vi "Pick Point.vi"(7 "Actual Transform In":T1, 8 "error in (no error)":errorcluster, 9 "Coords":cluster{"Horizontal":i32, "Vertical":i32}, 10 "Vertex Array":cluster{"X":sgl, "Y":sgl, "Z":sgl}[](array[cluster]), 11 "3D Picture Control In":refnum<vi>) -> (0 "error out":errorcluster, 1 "Hit Any Point?":bool, 2 "Snap Cursor Position":cluster{"X":sgl, "Y":sgl, "Z":sgl}, 3 "3D Picture Control Out":refnum<vi>, 5 "Actual Transform Out":T1)   [LabVIEW 2020, in "3D Plot.lvclass"]
uses:
  3D Plot.lvclass
  Actual Transform.ctl
  Range Clusters.ctl
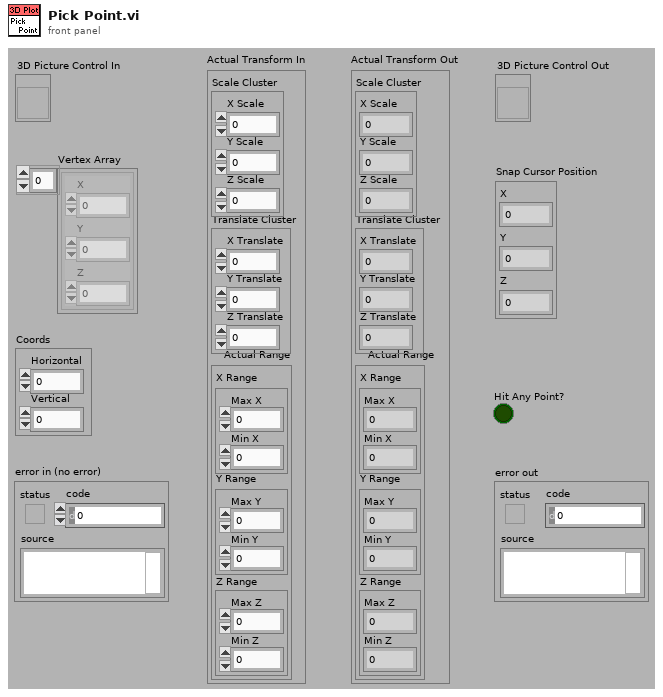
[diagram p1: front panel]
types:
  T1 = typedef "3D Plot.lvclass/Actual Transform.ctl" = cluster{"Scale Cluster":cluster{"X Scale":sgl, "Y Scale":sgl, "Z Scale":sgl}, "Translate Cluster":cluster{"X Translate":sgl, "Y Translate":sgl, "Z Translate":sgl}, "Actual Range":T2}
  T2 = typedef "3D Plot.lvclass/Range Clusters.ctl" = cluster{"X Range":cluster{"Max X":sgl, "Min X":sgl}, "Y Range":cluster{"Max Y":sgl, "Min Y":sgl}, "Z Range":cluster{"Max Z":sgl, "Min Z":sgl}}
  T3 = cluster{"Real Matrix Element":sgl, "Real Matrix Element":sgl, "Real Matrix Element":sgl}[]
  T4 = cluster{"Real Matrix Element":sgl, "Real Matrix Element":sgl, "Real Matrix Element":sgl}
  T5 = typedef "LVPoint32TypeDef.ctl" = cluster{"Horizontal":i32, "Vertical":i32}
  T6 = typedef "LVBoundsTypeDef.ctl" = cluster{"Width":u32, "Height":u32}
  T7 = cluster{"Product[0]":sgl, "Product[1]":sgl, "Product[2]":sgl}
  T8 = cluster{"X Translate":sgl, "Y Translate":sgl, "Z Translate":sgl}
  T9 = cluster{"X Scale":sgl, "Y Scale":sgl, "Z Scale":sgl}
  T10 = cluster{cluster{"Product[0]":sgl, "Product[1]":sgl, "Product[2]":sgl}, cluster{"Product[0]":sgl, "Product[1]":sgl, "Product[2]":sgl}}
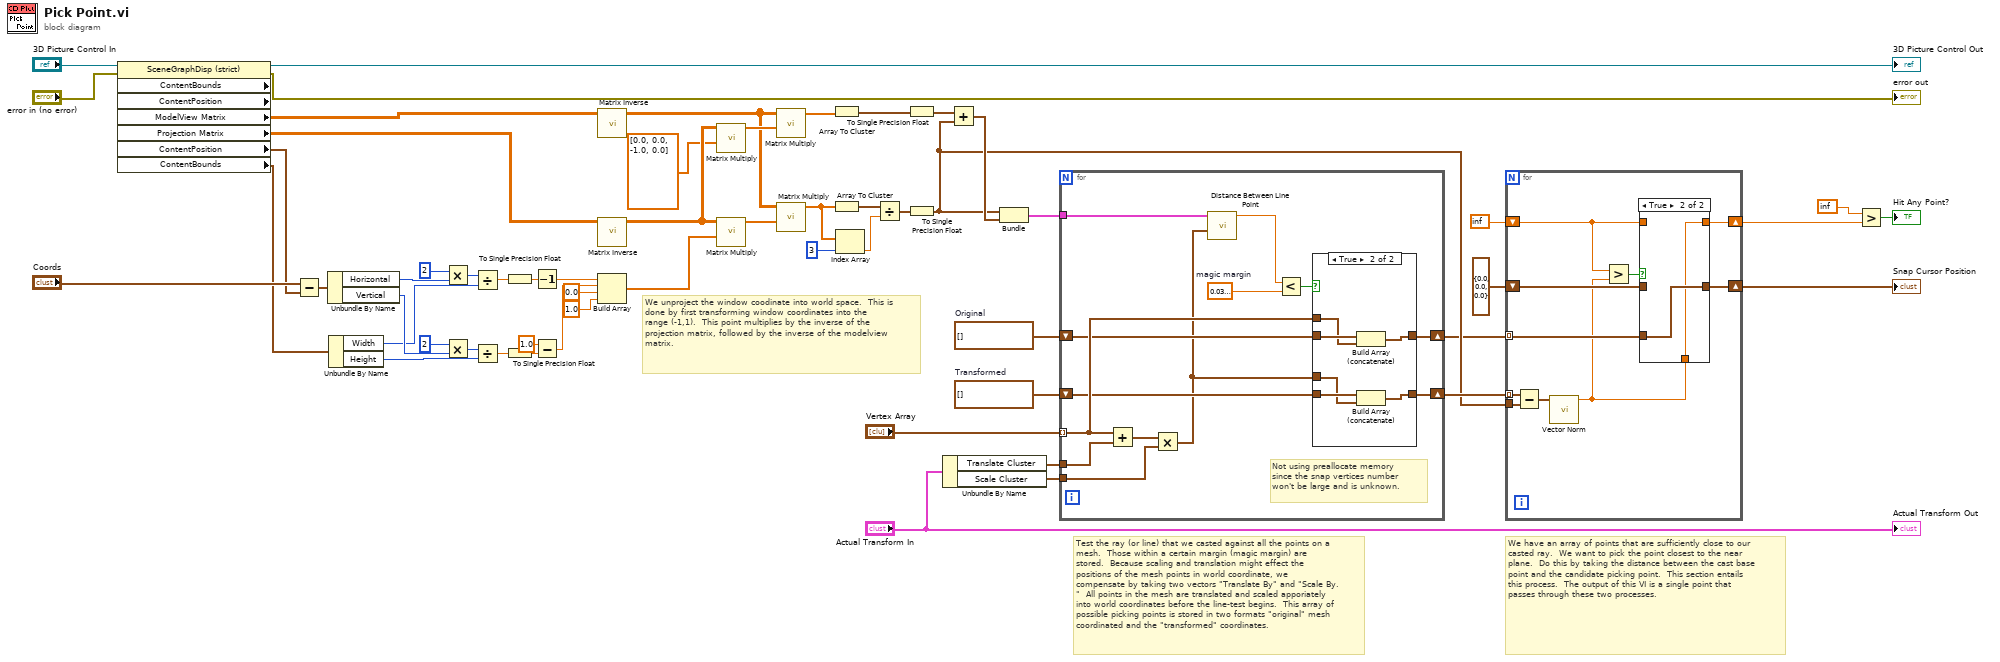
[diagram p0: block diagram]
diagram:
  w41 = T3 []  # Transformed
  w42 = T3 []  # Original
  # "We have an array of points that are sufficiently close to our casted ray.  We want to pick the point closest to the near plane.  Do this by taking the distance between the cast base point and the candidate picking point.  This section entails this process.  The output of this VI is a single point that passes through these two processes."
  # "Test the ray (or line) that we casted against all the points on a mesh.  Those within a certain margin (magic margin) are stored.  Because scaling and translation might effect the positions of the mesh points in world coordinate, we compensate by taking two vectors \"Translate By\" and \"Scale By.\"  All points in the mesh are translated and scaled apporiately into world coordinates before the line-test begins.  This array of possible picking points is stored in two formats \"original\" mesh coordinated and the \"transformed\" coordinates."
  # "We unproject the window coodinate into world space.  This is done by first transforming window coordinates into the range (-1,1).  This point multiplies by the inverse of the projection matrix, followed by the inverse of the modelview matrix."
  n1 = property on="Property Node" class="SceneGraphDisp (strict)" props=["ContentBounds", "ContentPosition", "ModelView Matrix", "Projection Matrix", "ContentPosition", "ContentBounds"](reference="3D Picture Control In", error in="error in (no error)") -> (reference out=→"3D Picture Control Out":refnum<vi>, error out=→"error out":errorcluster, "ModelView Matrix"=w11:sgl[][], "Projection Matrix"=w10:sgl[][], "ContentPosition"=w3:T5, "ContentBounds"=w2:T6)  [unwired: 2 out]
  n2 = Subtract(x="Coords", y=w3) -> (x-y=w8:T5)
  n3 = Unbundle By Name(w8) -> ("Horizontal"=w32:i32, "Vertical"=w31:i32)
  n4 = Unbundle By Name(w2) -> ("Width"=w30:u32, "Height"=w29:u32)
  n5 = Multiply(x=2 ("y"), y=w32) -> (x*y=w57:i32)
  n6 = Multiply(x=2 ("y"), y=w31) -> (x*y=w55:i32)
  n7 = Divide(x=w57, y=w30) -> (x/y=w56:dbl)
  n8 = Divide(x=w55, y=w29) -> (x/y=w47:dbl)
  n9 = To Single Precision Float(number=w56) -> (single precision float=w19:sgl)
  n10 = To Single Precision Float(number=w47) -> (single precision float=w20:sgl)
  n11 = Decrement(x=w19) -> (x-1=w48:sgl)
  n12 = Subtract(x=sgl 1.0, y=w20) -> (x-y=w46:sgl)
  n13 = call "Matrix Inverse.vi"("A"=w11) -> ("Inverse A"=w13:sgl[][])  [unwired: 10 out]
  n14 = call "Matrix Inverse.vi"("A"=w10) -> ("Inverse A"=w18:sgl[][])  [unwired: 10 out]
  n15 = Build Array(w48, w46, sgl 0.0 ("x"), sgl 1.0 ("element")) -> (w21:sgl[])
  n16 = call "Matrix Multiply.vi"("Vector"=sgl[] [0.0, 0.0, -1.0, 0.0], "Matrix"=w18) -> ("Product"=w14:sgl[])  [unwired: 9 out]
  n17 = call "Matrix Multiply.vi"("Vector"=w21, "Matrix"=w18) -> ("Product"=w16:sgl[])  [unwired: 9 out]
  n18 = call "Matrix Multiply.vi"("Vector"=w14, "Matrix"=w13) -> ("Product"=w15:sgl[])  [unwired: 9 out]
  n19 = call "Matrix Multiply.vi"("Vector"=w16, "Matrix"=w13) -> ("Product"=w17:sgl[])  [unwired: 9 out]
  n20 = Array To Cluster(array=w15) -> (cluster=w25:T7)
  n21 = Array To Cluster(array=w17) -> (cluster=w52:T7)
  n22 = Index Array(array=w17, index=3) -> (element=w51:sgl)
  n23 = Divide(x=w52, y=w51) -> (x/y=w23:T7)
  n24 = To Single Precision Float(number=w25) -> (single precision float=w24:T7)
  n25 = To Single Precision Float(number=w23) -> (single precision float=w22:T7)
  n26 = Unbundle By Name("Actual Transform In") -> ("Translate Cluster"=w28:T8, "Scale Cluster"=w27:T9)
  n27 = Add(x=w24, y=w22) -> (x+y=w44:T7)
  n28 = Bundle(w22, w44) -> (w43:T10)  [unwired: 1 out]
  n29 = for {
    tunnel: "Vertex Array" -> [w66] mode=indexing
    tunnel: w27 -> [w68]
    tunnel: w28 -> [w69]
    tunnel: w43 -> [w61]
    shift-right: [w63] -> w1
    shift-left: w42 -> [w65]
    shift-right: [w62] -> w40
    shift-left: w41 -> [w64]
    w67 = sgl 0.04  # magic margin
    # "Not using preallocate memory\nsince the snap vertices number\nwon't be large and is unknown."
    n30 = Add(x=w66, y=w69) -> (x+y=w70:cluster{sgl, sgl, sgl})
    n31 = Multiply(x=w70, y=w68) -> (x*y=w60:cluster{sgl, sgl, sgl})
    n32 = call "Distance Between Line Point.vi"("Point"=w60, "Line"=w61) -> ("Distance"=w59:sgl)  [unwired: 9 out]
    n33 = Less?(x=w59, y=w67) -> (x < y?=w71:bool)
    n34 = case shown="True" w71 {
      tunnel: w66 -> [_ w78]
      tunnel: w65 -> [w73 w79]
      tunnel: w60 -> [_ w75]
      tunnel: w64 -> [w72 w76]
      tunnel: [w73 w77] -> w63
      tunnel: [w72 w74] -> w62
      frame False {
      }
      frame True {
        n35 = Build Array (concatenate)(w79, w78) -> (w77:cluster{"X":sgl, "Y":sgl, "Z":sgl}[])
        n36 = Build Array (concatenate)(w76, w75) -> (w74:T3)
      }
    }
  }
  n37 = for {
    tunnel: w1 -> [w82] mode=indexing
    tunnel: w40 -> [w89] mode=indexing
    shift-right: [w85] -> w35
    shift-left: T4 {"Real Matrix Element"=0.0, "Real Matrix Element"=0.0, "Real Matrix Element"=0.0} -> [w86]
    shift-right: [w83] -> w37
    shift-left: sgl inf -> [w84]
    tunnel: w22 -> [w88]
    n38 = Subtract(x=w89, y=w88) -> (x-y=w81:cluster{sgl, sgl, sgl})
    n39 = call "Vector Norm.vi"("Vector"=w81) -> ("Norm"=w80:sgl)  [unwired: 10 out]
    n40 = Greater?(x=w84, y=w80) -> (0:w87:bool)
    n41 = case shown="True" w87 {
      tunnel: w86 -> [w91 _]
      tunnel: [w91 w93] -> w85
      tunnel: w84 -> [w90 _]
      tunnel: [w90 w92] -> w83
      tunnel: w82 -> [_ w93]
      tunnel: w80 -> [_ w92]
      frame False {
      }
      frame True {
      }
    }
  }
  "Snap Cursor Position" <- w35
  n42 = Greater?(x=sgl inf, y=w37) -> (0:→"Hit Any Point?":bool)
  "Actual Transform Out" <- "Actual Transform In"
